vi "datahandle.vi"(0 "object in":refnum<class "serial_work.lvclass">, 1 "字符串":string, 5 "error in (no error)":errorcluster) -> (14 "object out":refnum<class "serial_work.lvclass">, 15 "命令编码CN":string, 16 "时间QN":string, 17 "数据":string, 18 "布尔":bool, 19 "error out":errorcluster)   [LabVIEW 2016, in "serial_work.lvclass"]
uses:
  serial_work.lvclass
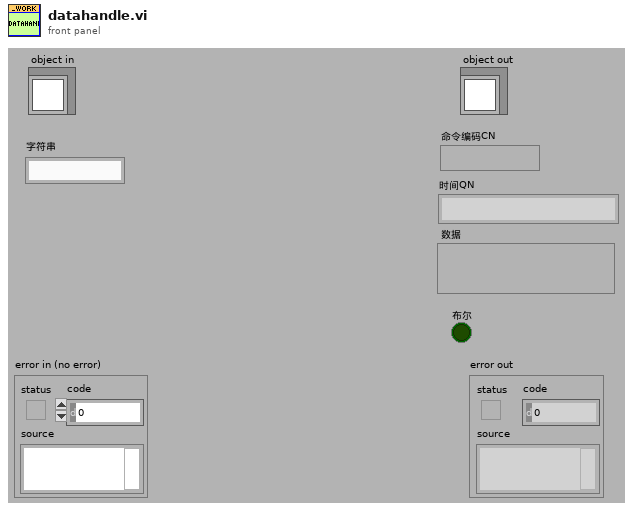
[diagram p1: front panel]
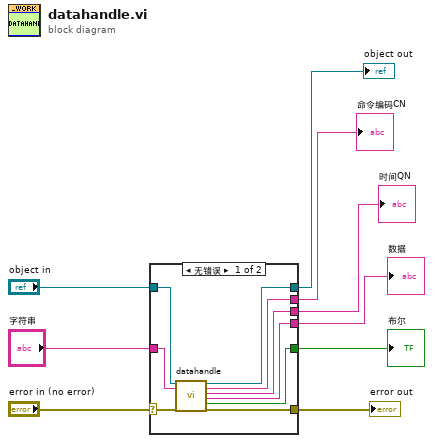
[diagram p0: block diagram]
diagram:
  n1 = case shown="无错误" "error in (no error)" {
    selector: "error in (no error)" -> [w16 w20]
    tunnel: [w15 w20] -> w8
    tunnel: [w17 w19] -> w6
    tunnel: "object in" -> [w18 w19]
    tunnel: "字符串" -> [w14 _]
    tunnel: [w13 _] -> w4
    tunnel: [w12 _] -> w3
    tunnel: [w11 _] -> w2
    tunnel: [w10 _] -> w1
    frame No Error {
      n2 = call-dynamic "datahandle.vi"("object in"=w18, "字符串"=w14, "error in (no error)"=w16) -> ("object out"=w17:refnum<class "serial_work.lvclass">, "命令编码CN"=w13:string, "时间QN"=w12:string, "数据"=w11:string, "布尔"=w10:bool, "error out"=w15:errorcluster)  [unwired: 11 in]
    }
    frame Error {
    }
  }
  "error out" <- w8
  "object out" <- w6
  "布尔" <- w1
  "数据" <- w2
  "时间QN" <- w3
  "命令编码CN" <- w4
